vi "Get_Status_BarcodeString_2.0.vi"(4 "error in (no error)":errorcluster, 7 "Data":T1={"Camera 1"={"Camera1"="", "Cam 1"=FALSE, "CAM1 Model"=enum."a2A5328-15ucBAS", "Cam1 ID"=0}, "Camera 2"={"Camera2"="", "Cam 2"=FALSE, "CAM2 Model"=enum."a2A5328-15ucBAS", "Cam2 ID"=0}, "Image"={"Camera1_Img"=refnum, "Camera2_Img"=refnum, "Img1_Orig_Disp"=refnum, "Img2_Orig_Disp"=refnum, "Img1_Orig_RGB"=refnum, "Img2_Orig_RGB"=refnum, "Blue_Plane_Extract"=refnum, "Subtracted_Plane"=refnum, "Img1_Binary"=refnum, "Img2_Binary"=refnum, "Crop_Mask"=refnum, "Img1_Save"=refnum, "Img2_Save"=refnum, "Img1_Cali_Full"=refnum, "Img2_Cali_Full"=refnum, "Img1_Cali_Detect"=refnum, "Img2_Cali_Detect"=refnum}, "Ques"={"Cam 1 queue"=refnum, "Cam 2 queue"=refnum, "Cam 1 - save queue"=refnum, "Cam 2 - save queue"=refnum, "Image Process Queue Size"=500, "Image Save Queue Size"=500, "Overload threshold"=500, "Max large object threshold"=0}, "Arduino SRS"={"Pinch-valve"="", "Actuator"=FALSE, "Open(T)/Close(F)"=FALSE, "Arduino Uno"=""}, "Pump"={"Port"="", "Connection"=FALSE, "Flush Size"=0, "Command"="", "Pump Size"=enum."None", "Pump"="", "Ready"=FALSE}, "Camera settings"={"Detection settings"={"Sample size threshold"=500, "Detection Region %"=30.0, "Timeout Sample"=200}, "Lens/camera settings"={"Aperture"=enum."Item 0", "Legacy Cam Attributes"=FALSE, "Max Framerate"=100, "Exposure Time"=1000.0, "Framerate"=15}, "Crop settings"={"Cam1"={"Rectangle 1"={"Left"=0, "Top"=0, "Right"=0, "Bottom"=0, "Rotation"=0.0}, "Camera Orientation 1"="", "Pixel to mm 1"=0.0}, "Cam2"={"Rectangle 2"={"Left"=0, "Top"=0, "Right"=0, "Bottom"=0, "Rotation"=0.0}, "Camera Orientation 2"="", "Pixel to mm 2"=0.0}}}, "Arduino ISS"={"Mega F3"="", "Phase3"=FALSE, "Barcode"="", "Sorting sys."=FALSE, "Initial size"=0.0, "Size Interval"=0.0, "Mun. of containers"=0.0, "Container nr."=0.0, "Arduino Mega"=""}, "Img_Capt"=FALSE, "Empty_Refill"=FALSE, "I don't think is in use"={"Light intensity"=100}, "Extended setup"={"Location"="Station", "Latitude"="Station", "Longitude"="Station", "Determiner"="Station", "Sex"="Station", "Station"="", "Collection date"=""}, "Main interface"={"Sample Name"="Test Sample", "Operator"="JFR", "Species Name"="", "Other Notes"=""}, "Tap1"=0, "SystemVersion"=0, "System Serial"="", "Exit"=FALSE, "Kuvette Full"=FALSE, "Core JKI"={"Current VI Reference"=refnum, "Close Panel on Exit?"=FALSE}, "Calibration"={"Calibration 1"=path "C:/Users/au540322/Desktop/IHS_Project/images/Debris/Debris_0/Debris_0_2019_06_01-23-32-49-686.PNG", "Calibration 2"=path "C:/Users/au540322/Desktop/IHS_Project/images/Debris/Debris_0/Debris_0_2019_06_01-23-32-49-686.PNG", "Detect 1"=path "C:/Users/au540322/Desktop/IHS_Project/images/Debris/Debris_0/Debris_0_2019_06_01-23-32-49-686.PNG", "Detect 2"=path "C:/Users/au540322/Desktop/IHS_Project/images/Debris/Debris_0/Debris_0_2019_06_01-23-32-49-686.PNG"}, "Auto Flush"=FALSE} {"SystemVersion" items=["Standard", "XL"]; "Tap1" items=["Session Data", "Extended Setup", "Buffer", "Camera", "Dispenser", "Stats", "Connections"]; "I don't think is in use"."Light intensity" scale=0.0..100.0; "Camera settings"."Crop settings"."Cam2"."Rectangle 2"."Rotation" format="%.2f"; "Camera settings"."Crop settings"."Cam2"."Rectangle 2"."Left" scale=0.0..1024.0; "Camera settings"."Crop settings"."Cam2"."Rectangle 2"."Right" scale=0.0..1024.0; "Camera settings"."Crop settings"."Cam1"."Rectangle 1"."Rotation" format="%.2f"; "Camera settings"."Crop settings"."Cam1"."Rectangle 1"."Left" scale=0.0..1024.0; "Camera settings"."Crop settings"."Cam1"."Rectangle 1"."Right" scale=0.0..1024.0; "Camera settings"."Lens/camera settings"."Framerate" min=1; "Camera settings"."Lens/camera settings"."Max Framerate" min=1; "Camera settings"."Detection settings"."Sample size threshold" min=1; "Pump"."Flush Size" min=0 max=6000 step=100; "Ques"."Overload threshold" min=1; "Ques"."Image Save Queue Size" min=1; "Ques"."Image Process Queue Size" min=1}) -> (0 "error out":errorcluster, 1 "F3 Status":string, 2 "VISA resource name out":refnum<visa-resource-name>, 3 "Data 2":T1={"Camera 1"={"Camera1"="", "Cam 1"=FALSE, "CAM1 Model"=enum."a2A5328-15ucBAS", "Cam1 ID"=0}, "Camera 2"={"Camera2"="", "Cam 2"=FALSE, "CAM2 Model"=enum."a2A5328-15ucBAS", "Cam2 ID"=0}, "Image"={"Camera1_Img"=refnum, "Camera2_Img"=refnum, "Img1_Orig_Disp"=refnum, "Img2_Orig_Disp"=refnum, "Img1_Orig_RGB"=refnum, "Img2_Orig_RGB"=refnum, "Blue_Plane_Extract"=refnum, "Subtracted_Plane"=refnum, "Img1_Binary"=refnum, "Img2_Binary"=refnum, "Crop_Mask"=refnum, "Img1_Save"=refnum, "Img2_Save"=refnum, "Img1_Cali_Full"=refnum, "Img2_Cali_Full"=refnum, "Img1_Cali_Detect"=refnum, "Img2_Cali_Detect"=refnum}, "Ques"={"Cam 1 queue"=refnum, "Cam 2 queue"=refnum, "Cam 1 - save queue"=refnum, "Cam 2 - save queue"=refnum, "Image Process Queue Size"=500, "Image Save Queue Size"=500, "Overload threshold"=500, "Max large object threshold"=0}, "Arduino SRS"={"Pinch-valve"="", "Actuator"=FALSE, "Open(T)/Close(F)"=FALSE, "Arduino Uno"=""}, "Pump"={"Port"="", "Connection"=FALSE, "Flush Size"=0, "Command"="", "Pump Size"=enum."None", "Pump"="", "Ready"=FALSE}, "Camera settings"={"Detection settings"={"Sample size threshold"=500, "Detection Region %"=30.0, "Timeout Sample"=200}, "Lens/camera settings"={"Aperture"=enum."Item 0", "Legacy Cam Attributes"=FALSE, "Max Framerate"=100, "Exposure Time"=1000.0, "Framerate"=15}, "Crop settings"={"Cam1"={"Rectangle 1"={"Left"=0, "Top"=0, "Right"=0, "Bottom"=0, "Rotation"=0.0}, "Camera Orientation 1"="", "Pixel to mm 1"=0.0}, "Cam2"={"Rectangle 2"={"Left"=0, "Top"=0, "Right"=0, "Bottom"=0, "Rotation"=0.0}, "Camera Orientation 2"="", "Pixel to mm 2"=0.0}}}, "Arduino ISS"={"Mega F3"="", "Phase3"=FALSE, "Barcode"="", "Sorting sys."=FALSE, "Initial size"=0.0, "Size Interval"=0.0, "Mun. of containers"=0.0, "Container nr."=0.0, "Arduino Mega"=""}, "Img_Capt"=FALSE, "Empty_Refill"=FALSE, "I don't think is in use"={"Light intensity"=100}, "Extended setup"={"Location"="Station", "Latitude"="Station", "Longitude"="Station", "Determiner"="Station", "Sex"="Station", "Station"="", "Collection date"=""}, "Main interface"={"Sample Name"="Test Sample", "Operator"="JFR", "Species Name"="", "Other Notes"=""}, "Tap1"=0, "SystemVersion"=0, "System Serial"="", "Exit"=FALSE, "Kuvette Full"=FALSE, "Core JKI"={"Current VI Reference"=refnum, "Close Panel on Exit?"=FALSE}, "Calibration"={"Calibration 1"=path "C:/Users/au540322/Desktop/IHS_Project/images/Debris/Debris_0/Debris_0_2019_06_01-23-32-49-686.PNG", "Calibration 2"=path "C:/Users/au540322/Desktop/IHS_Project/images/Debris/Debris_0/Debris_0_2019_06_01-23-32-49-686.PNG", "Detect 1"=path "C:/Users/au540322/Desktop/IHS_Project/images/Debris/Debris_0/Debris_0_2019_06_01-23-32-49-686.PNG", "Detect 2"=path "C:/Users/au540322/Desktop/IHS_Project/images/Debris/Debris_0/Debris_0_2019_06_01-23-32-49-686.PNG"}, "Auto Flush"=FALSE} {"SystemVersion" items=["Standard", "XL"]; "Tap1" items=["Session Data", "Extended Setup", "Buffer", "Camera", "Dispenser", "Stats", "Connections"]; "I don't think is in use"."Light intensity" scale=0.0..100.0; "Camera settings"."Crop settings"."Cam2"."Rectangle 2"."Rotation" format="%.2f"; "Camera settings"."Crop settings"."Cam2"."Rectangle 2"."Left" scale=0.0..1024.0; "Camera settings"."Crop settings"."Cam2"."Rectangle 2"."Right" scale=0.0..1024.0; "Camera settings"."Crop settings"."Cam1"."Rectangle 1"."Rotation" format="%.2f"; "Camera settings"."Crop settings"."Cam1"."Rectangle 1"."Left" scale=0.0..1024.0; "Camera settings"."Crop settings"."Cam1"."Rectangle 1"."Right" scale=0.0..1024.0; "Camera settings"."Lens/camera settings"."Framerate" min=1; "Camera settings"."Lens/camera settings"."Max Framerate" min=1; "Camera settings"."Detection settings"."Sample size threshold" min=1; "Pump"."Flush Size" min=0 max=6000 step=100; "Ques"."Overload threshold" min=1; "Ques"."Image Save Queue Size" min=1; "Ques"."Image Process Queue Size" min=1})   [LabVIEW 2024]
uses:
  controls/Data_JKI.ctl
  <vilib>/userDefined/High Color/IMAQdx.ctl
  <vilib>/vision/Image Controls.llb/IMAQ Image.ctl
  ae539422-90c2-48c7-a089-5bb01302e7c9.vi
  d7fcdf58-1d6e-4c9b-b4c1-69249527c4a7.vi
  644cd9a0-6467-4848-a5d8-4a56f541d81a.vi
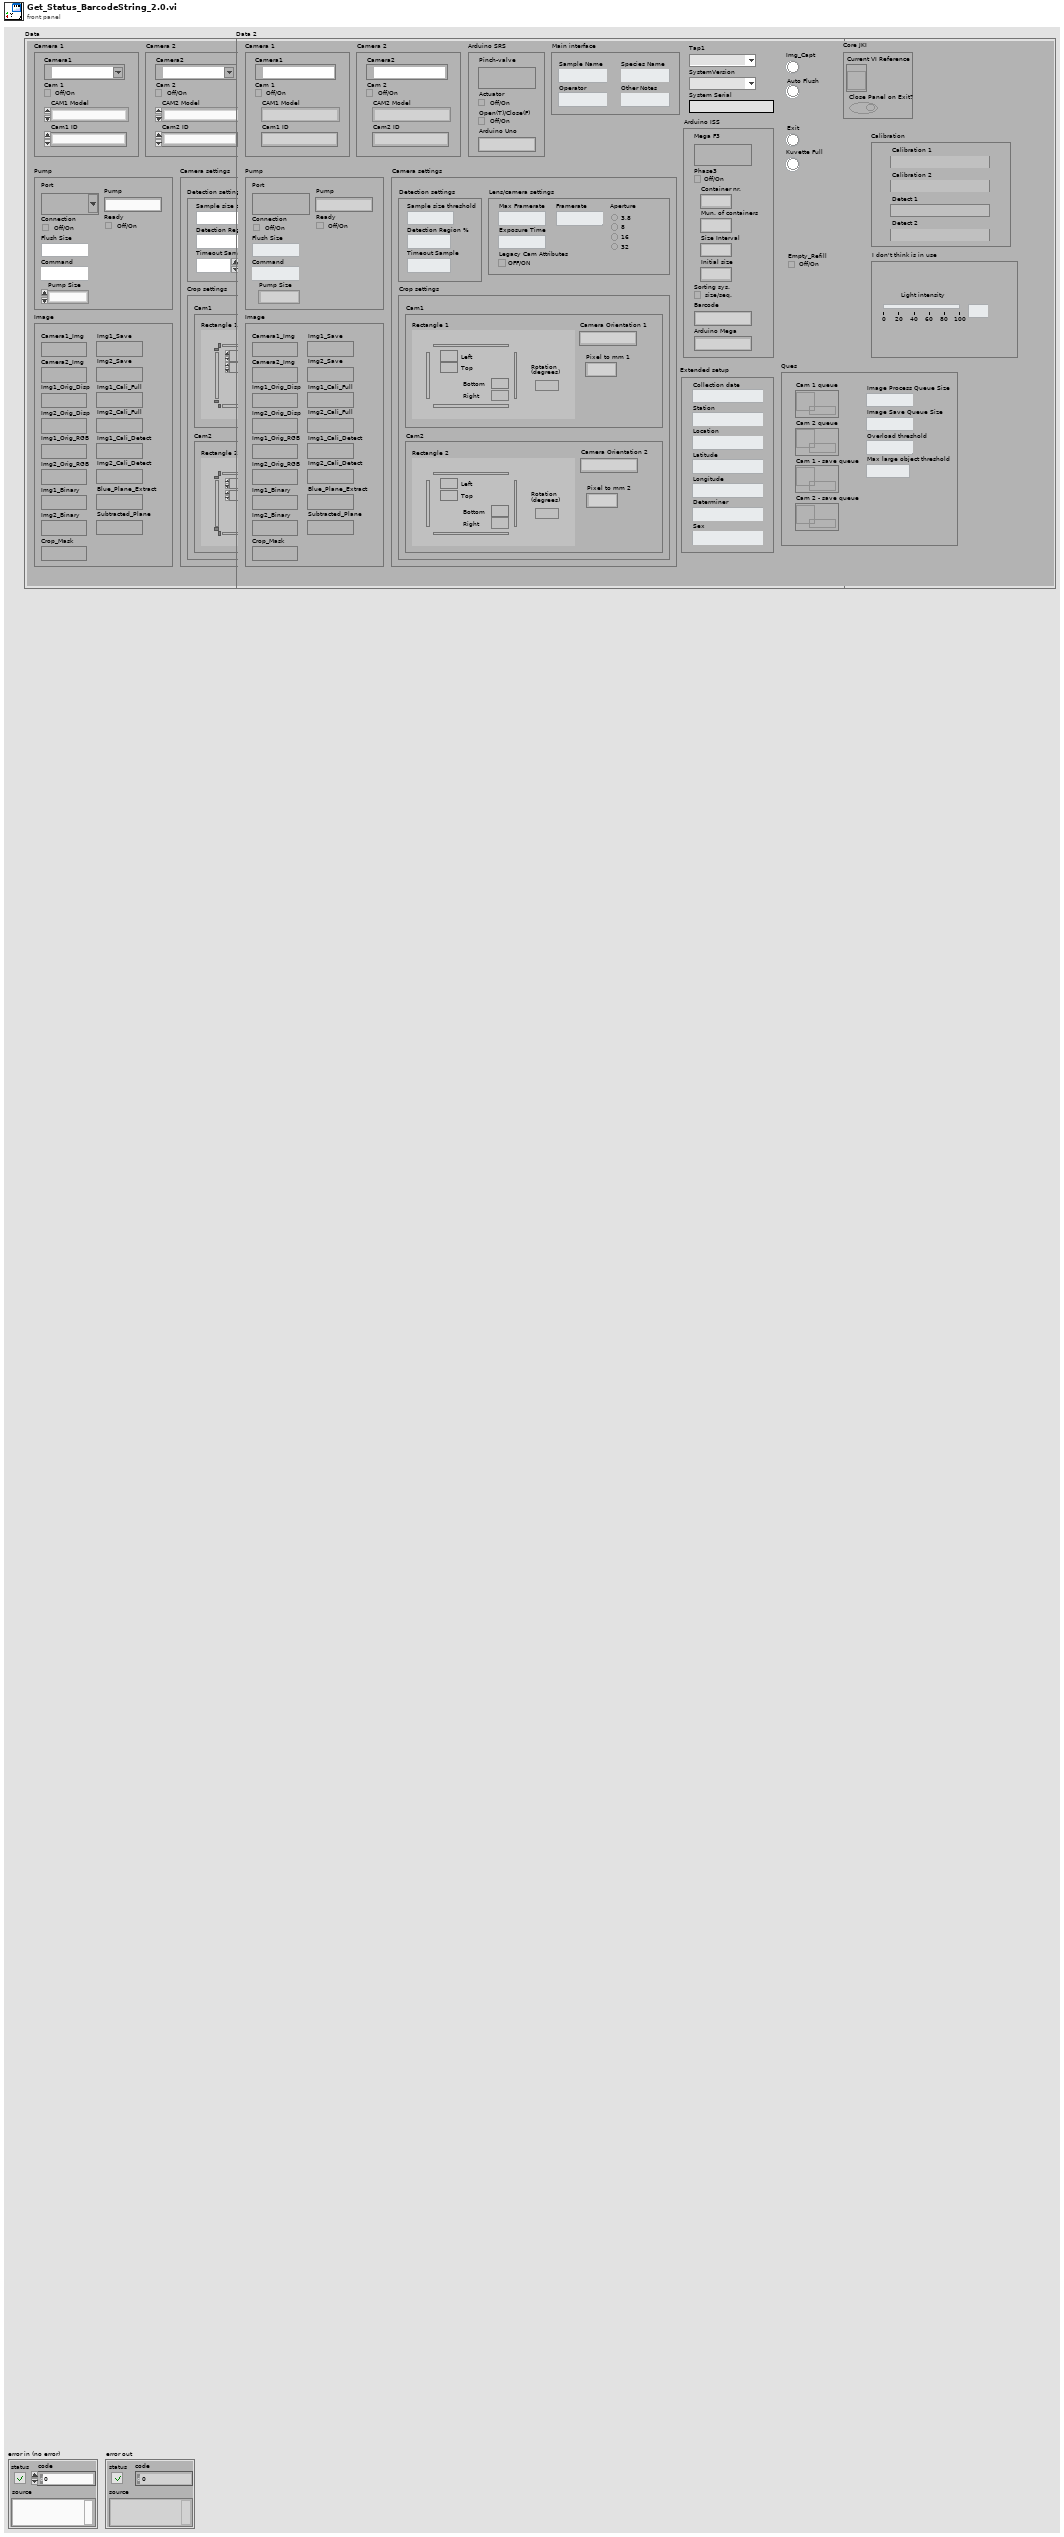
[diagram p1: front panel]
types:
  T1 = typedef "Data_JKI.ctl" = cluster{"Camera 1":cluster{"Camera1":T2, "Cam 1":bool, "CAM1 Model":enum16{"a2A5328-15ucBAS", "acA1920-155uc"}, "Cam1 ID":i32}, "Camera 2":cluster{"Camera2":T2, "Cam 2":bool, "CAM2 Model":enum16{"a2A5328-15ucBAS", "acA1920-155uc"}, "Cam2 ID":i32}, "Image":cluster{"Camera1_Img":T3, "Camera2_Img":T3, "Img1_Orig_Disp":T3, "Img2_Orig_Disp":T3, "Img1_Orig_RGB":T3, "Img2_Orig_RGB":T3, "Blue_Plane_Extract":T3, "Subtracted_Plane":T3, "Img1_Binary":T3, "Img2_Binary":T3, "Crop_Mask":T3, "Img1_Save":T3, "Img2_Save":T3, "Img1_Cali_Full":T3, "Img2_Cali_Full":T3, "Img1_Cali_Detect":T3, "Img2_Cali_Detect":T3}, "Ques":cluster{"Cam 1 queue":refnum<queue>, "Cam 2 queue":refnum<queue>, "Cam 1 - save queue":refnum<queue>, "Cam 2 - save queue":refnum<queue>, "Image Process Queue Size":i32, "Image Save Queue Size":i32, "Overload threshold":i32, "Max large object threshold":i32}, "Arduino SRS":cluster{"Pinch-valve":refnum<visa-resource-name>, "Actuator":bool, "Open(T)/Close(F)":bool, "Arduino Uno":string}, "Pump":cluster{"Port":refnum<visa-resource-name>, "Connection":bool, "Flush Size":i32, "Command":string, "Pump Size":enum16{"None", "Small", "Large"}, "Pump":string, "Ready":bool}, "Camera settings":cluster{"Detection settings":cluster{"Sample size threshold":i32, "Detection Region %":dbl, "Timeout Sample":i32}, "Lens/camera settings":cluster{"Aperture":enum32{"Item 0", "Item 1", "Item 2", "Item 3"}, "Legacy Cam Attributes":bool, "Max Framerate":i32, "Exposure Time":dbl, "Framerate":i32}, "Crop settings":cluster{"Cam1":cluster{"Rectangle 1":T4, "Camera Orientation 1":string, "Pixel to mm 1":dbl}, "Cam2":cluster{"Rectangle 2":T4, "Camera Orientation 2":string, "Pixel to mm 2":dbl}}}, "Arduino ISS":cluster{"Mega F3":refnum<visa-resource-name>, "Phase3":bool, "Barcode":string, "Sorting sys.":bool, "Initial size":dbl, "Size Interval":dbl, "Mun. of containers":dbl, "Container nr.":dbl, "Arduino Mega":string}, "Img_Capt":bool, "Empty_Refill":bool, "I don't think is in use":cluster{"Light intensity":i32}, "Extended setup":cluster{"Location":string, "Latitude":string, "Longitude":string, "Determiner":string, "Sex":string, "Station":string, "Collection date":string}, "Main interface":cluster{"Sample Name":string, "Operator":string, "Species Name":string, "Other Notes":string}, "Tap1":u16, "SystemVersion":u16, "System Serial":string, "Exit":bool, "Kuvette Full":bool, "Core JKI":cluster{"Current VI Reference":refnum<vi>, "Close Panel on Exit?":bool}, "Calibration":cluster{"Calibration 1":path, "Calibration 2":path, "Detect 1":path, "Detect 2":path}, "Auto Flush":bool}
  T2 = typedef "IMAQdx.ctl" = refnum<k21>
  T3 = typedef "IMAQ Image.ctl" = refnum<image>
  T4 = typedef "IMAQ Rectangle" = cluster{"Left":i32, "Top":i32, "Right":i32, "Bottom":i32, "Rotation":dbl}
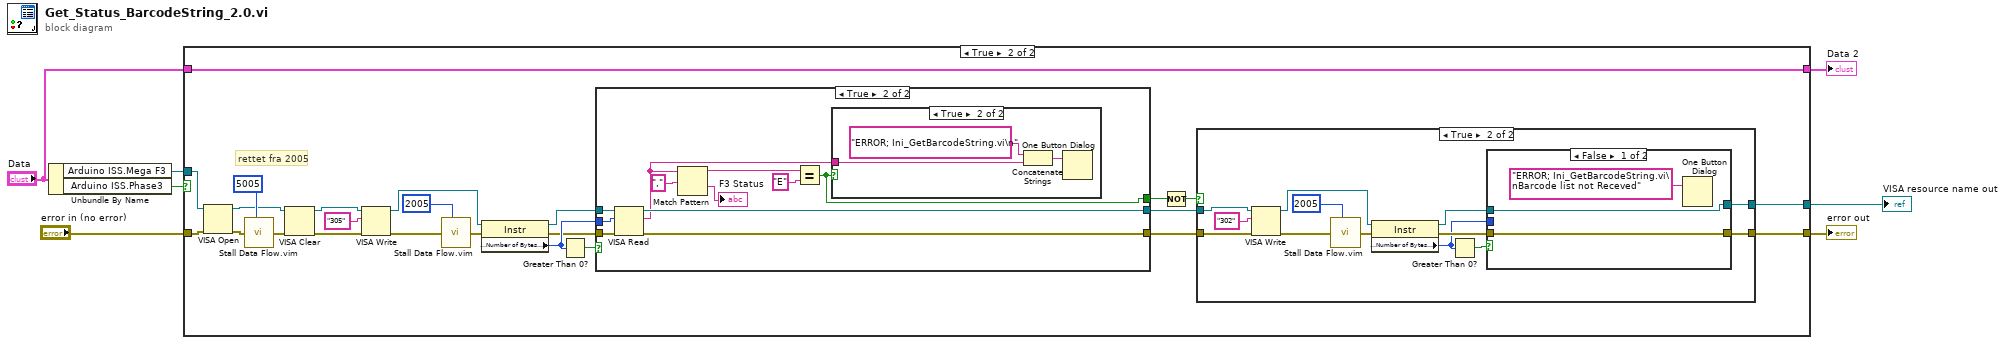
[diagram p0: block diagram]
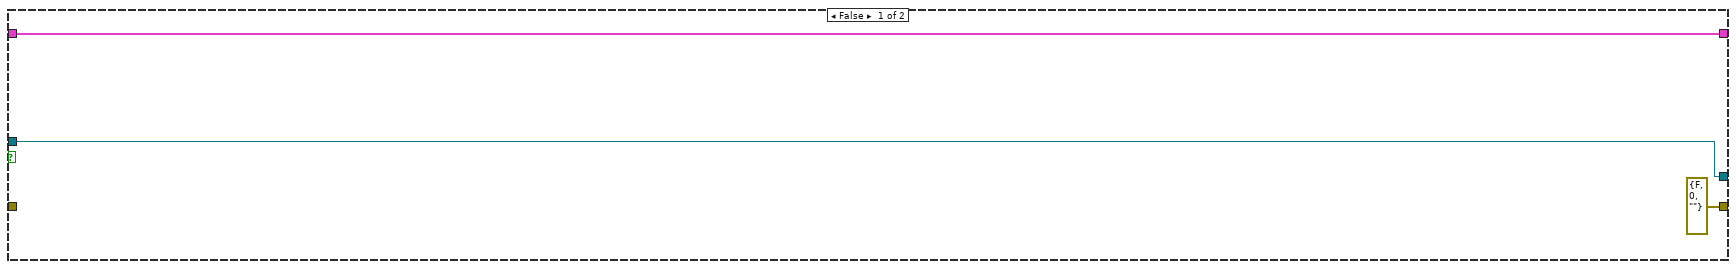
[diagram p2: hidden frame]
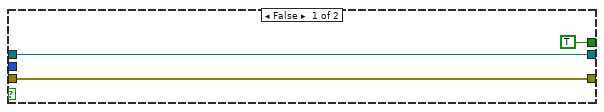
[diagram p3: hidden frame]
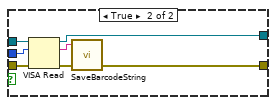
[diagram p6: hidden frame]
diagram:
  n1 = Unbundle By Name("Data") -> ("Arduino ISS.Mega F3"=w6:refnum<visa-resource-name>, "Arduino ISS.Phase3"=w7:bool)
  n2 = case shown="True" w7 {
    tunnel: "Data" -> [w10 w32]
    tunnel: [w10 w32] -> w1
    tunnel: [errorcluster {"status"=FALSE, "code"=0, "source"=""} ("error out") w34] -> w4
    tunnel: w6 -> [w8 w23]
    tunnel: "error in (no error)" -> [_ w19]
    tunnel: [w8 w11] -> w3
    frame False {
    }
    frame True {
      # "rettet fra 2005"
      n3 = VISA Open(error in (no error)=w19, VISA resource name=w23) -> (VISA resource name=w15:refnum<visa-resource-name>, error out=w18:errorcluster)  [unwired: 3 in]
      n4 = call "Stall Data Flow.vim"("value in"=w18, "milliseconds to wait"=u32 5005) -> ("value out"=w17:errorcluster)  [unwired: 1 out]
      n5 = VISA Clear(VISA resource name=w15, error in (no error)=w17) -> (VISA resource name out=w31:refnum<visa-resource-name>, error out=w16:errorcluster)
      n6 = VISA Write(VISA resource name=w31, write buffer="305", error in (no error)=w16) -> (VISA resource name out=w12:refnum<visa-resource-name>, error out=w14:errorcluster)  [unwired: 1 out]
      n7 = call "Stall Data Flow.vim"("value in"=w14, "milliseconds to wait"=u32 2005) -> ("value out"=w13:errorcluster)  [unwired: 1 out]
      n8 = property class="Instr"(reference=w12, error in=w13) -> (reference out=w28:refnum<visa-resource-name>, error out=w27:errorcluster, "Serial Settings:Number of Bytes at Serial Port"=w29:u32)
      n9 = Greater Than 0?(x=w29) -> (x > 0?=w30:bool)
      n10 = case shown="True" w30 {
        tunnel: w29 -> [_ w46]
        tunnel: w28 -> [w37 w48]
        tunnel: w27 -> [w36 w47]
        tunnel: [w37 w45] -> w33
        tunnel: [w36 w44] -> w20
        tunnel: [TRUE w40] -> w21
        frame False {
        }
        frame True {
          n11 = VISA Read(VISA resource name=w48, byte count=w46, error in (no error)=w47) -> (VISA resource name out=w45:refnum<visa-resource-name>, read buffer=w39:string, error out=w44:errorcluster)  [unwired: 1 out]
          n12 = Match Pattern(string=w39, regular expression=",") -> (before substring=w41:string, after substring=→"F3 Status":string)  [unwired: 1 in, 2 out]
          n13 = Equal?(x=w41, y="E") -> (x = y?=w40:bool)
          n14 = case shown="True" w40 {
            tunnel: w39 -> [_ w49]
            frame False {
            }
            frame True {
              n15 = Concatenate Strings("ERROR; Ini_GetBarcodeString.vi\n", w49) -> (w50:string)
              n16 = One Button Dialog(message=w50) -> ()  [unwired: 1 in, 1 out]
            }
          }
        }
      }
      n17 = Not(x=w21) -> (.not. x?=w24:bool)
      n18 = case shown="True" w24 {
        tunnel: [w53 w62] -> w34
        tunnel: w33 -> [w52 w54]
        tunnel: w20 -> [w53 w55]
        tunnel: [w52 w56] -> w11
        frame False {
        }
        frame True {
          n19 = VISA Write(VISA resource name=w54, write buffer="302", error in (no error)=w55) -> (VISA resource name out=w57:refnum<visa-resource-name>, error out=w59:errorcluster)  [unwired: 1 out]
          n20 = call "Stall Data Flow.vim"("value in"=w59, "milliseconds to wait"=u32 2005) -> ("value out"=w58:errorcluster)  [unwired: 1 out]
          n21 = property class="Instr"(reference=w57, error in=w58) -> (reference out=w64:refnum<visa-resource-name>, error out=w63:errorcluster, "Serial Settings:Number of Bytes at Serial Port"=w61:u32)
          n22 = Greater Than 0?(x=w61) -> (x > 0?=w65:bool)
          n23 = case shown="False" w65 {
            tunnel: w64 -> [w68 w76]
            tunnel: w63 -> [w67 w75]
            tunnel: [w67 w72] -> w62
            tunnel: w61 -> [_ w71]
            tunnel: [w68 w70] -> w56
            frame False {
              n24 = One Button Dialog(message="ERROR; Ini_GetBarcodeString.vi\nBarcode list not Receved") -> ()  [unwired: 1 in, 1 out]
            }
            frame True {
              n25 = VISA Read(VISA resource name=w76, byte count=w71, error in (no error)=w75) -> (VISA resource name out=w70:refnum<visa-resource-name>, read buffer=w74:string, error out=w73:errorcluster)  [unwired: 1 out]
              n26 = call "SaveBarcodeString.vi"("error in"=w73, "String"=w74) -> ("error out"=w72:errorcluster)  [unwired: 3 in]
            }
          }
        }
      }
    }
  }
  "error out" <- w4
  "VISA resource name out" <- w3
  "Data 2" <- w1
